vi "Remove too small lines.vi"(11 "All Lines":T1[](array[typedef])) -> (3 "Big Enough Lines":T1[](array[typedef]))   [LabVIEW 2017]
uses:
  Vector Library/Line.ctl
  Vector Library/Vector.ctl
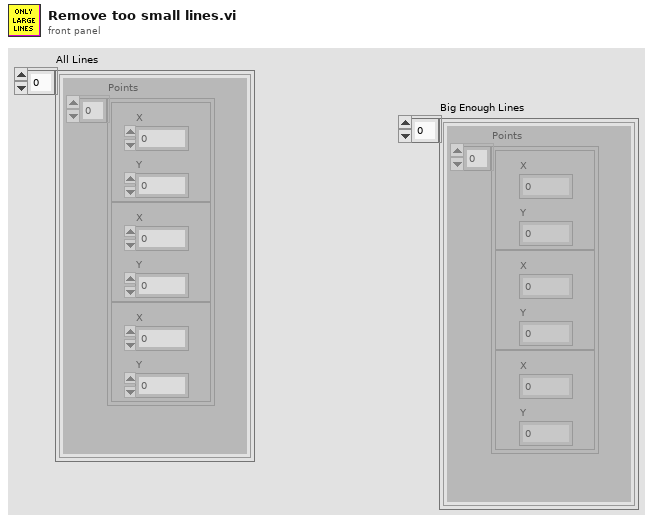
[diagram p1: front panel]
types:
  T1 = typedef "Line.ctl" = cluster{"Points":T2[]}
  T2 = typedef "Vector.ctl" = cluster{"X":dbl, "Y":dbl}
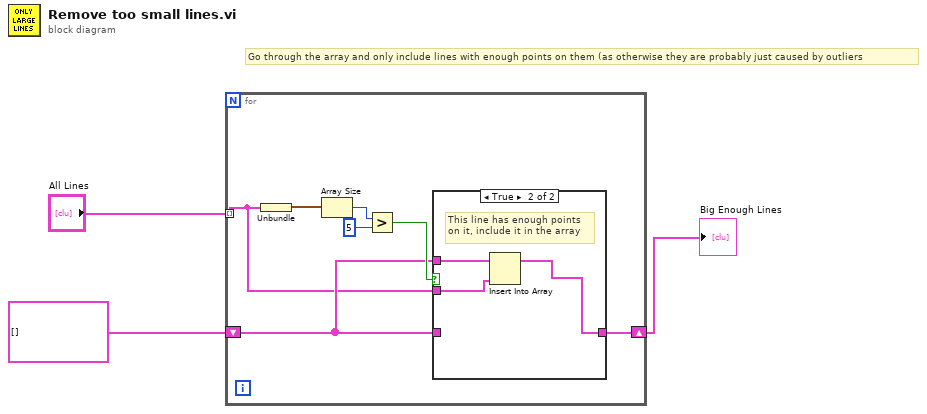
[diagram p0: block diagram]
diagram:
  # "Go through the array and only include lines with enough points on them (as otherwise they are probably just caused by outliers"
  n1 = for {
    shift-right: [w6] -> w2
    shift-left: cluster{"Points":cluster{"X":dbl, "Y":dbl}[]}[] [] ("Big Enough Lines") -> [w5]
    tunnel: "All Lines" -> [w4] mode=indexing
    n2 = Unbundle(w4) -> ("Points"=w10:T2[])
    n3 = Array Size(array=w10) -> (size(s)=w9:i32)
    n4 = Greater?(x=w9, y=5) -> (0:w7:bool)
    n5 = case shown="True" w7 {
      tunnel: [w11 w12] -> w6
      tunnel: w5 -> [w11 _]
      tunnel: w5 -> [_ w14]
      tunnel: w4 -> [_ w13]
      frame False {
        # "This line doesn't have\nenough points on it,\ndon't include it in the array"
      }
      frame True {
        # "This line has enough points\non it, include it in the array"
        n6 = Insert Into Array(array=w14, new element=w13) -> (w12:cluster{"Points":cluster{"X":dbl, "Y":dbl}[]}[])  [unwired: 1 in]
      }
    }
  }
  "Big Enough Lines" <- w2
